vi "Test Overlay Sector.vi"() -> ()   [LabVIEW 2013]
uses:
  Test Sector Cluster.ctl
panel:
  in  "All?":bool
  in  "Sector":u8=3
  out "Image":T1(plugin-control)
  in  "File Path":path
  in  "[Test Sectors]":T2[](array[typedef])=array[43543 elements]
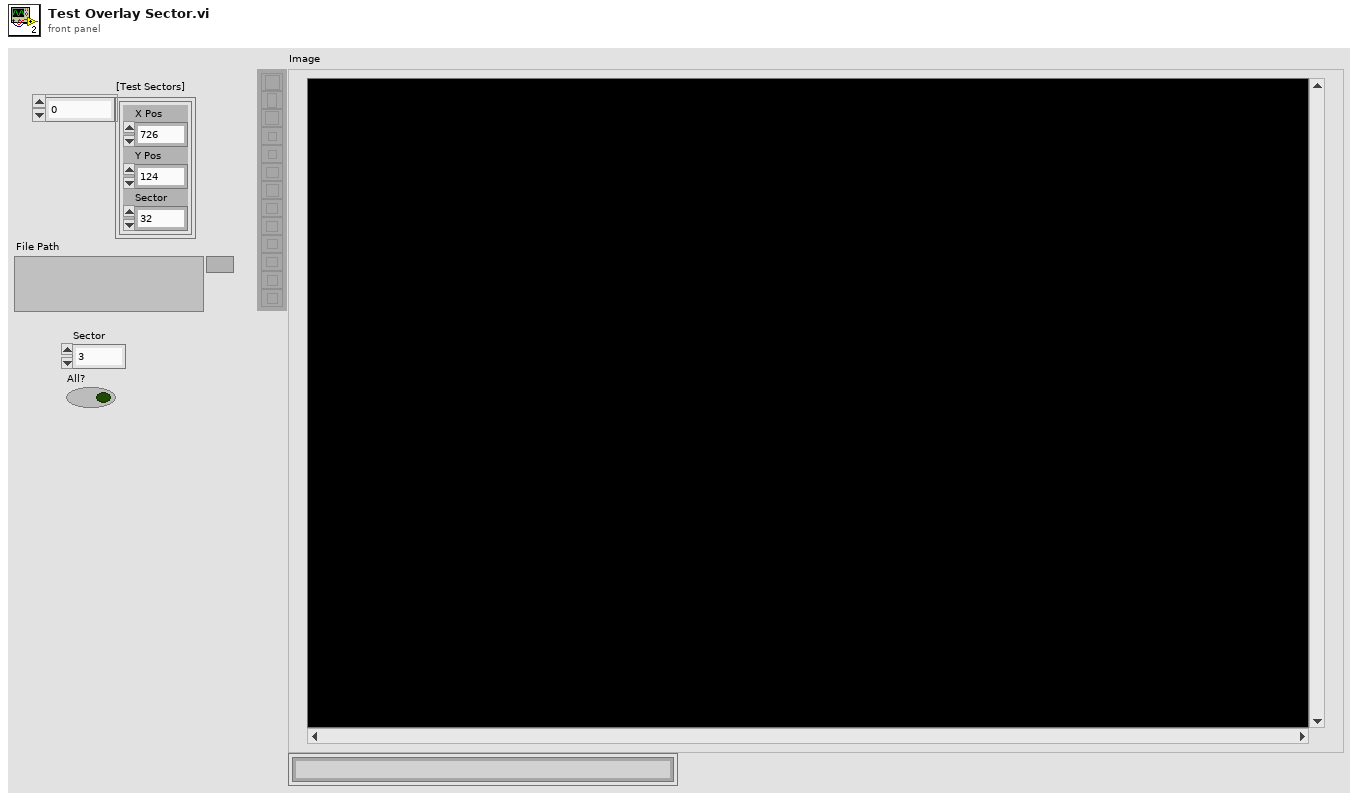
[diagram p1: front panel]
types:
  T1 = typedef "IMAQ Image.ctl" = refnum<image>
  T2 = typedef "Test Sector Cluster.ctl" = cluster{"X Pos":u16, "Y Pos":u16, "Sector":u8}
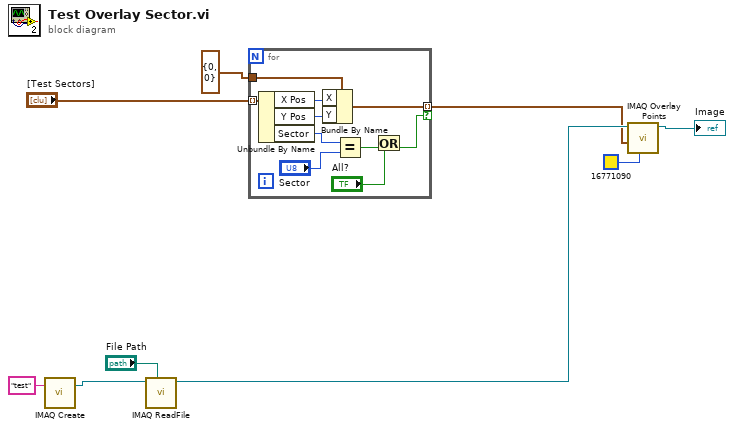
[diagram p0: block diagram]
diagram:
  n1 = call "IMAQ Create"("Image Name"="test") -> ("New Image"=w8:T1)  [unwired: 4 in, 1 out]
  n2 = call "IMAQ ReadFile"("File Path"="File Path", "Image"=w8) -> ("Image Out"=w5:T1)  [unwired: 5 in, 4 out]
  n3 = for {
    tunnel: cluster{"X":i32, "Y":i32} {"X"=0, "Y"=0} ("Point") -> [w19]
    tunnel: "[Test Sectors]" -> [w18] mode=indexing
    tunnel: [w15] -> w3 mode=indexing if=w11
    n4 = Unbundle By Name(w18) -> ("X Pos"=w17:u16, "Y Pos"=w16:u16, "Sector"=w14:u8)
    n5 = Bundle By Name(cluster=w19, "X"=w17, "Y"=w16) -> (w15:cluster{"X":i32, "Y":i32})
    n6 = Equal?(x=w14, y="Sector") -> (x = y?=w12:bool)
    n7 = Or(x="All?", y=w12) -> (x .or. y?=w11:bool)
  }
  n8 = call "IMAQ Overlay Points"("Color"=u32 16771090, "Array of Points"=w3, "Image"=w5) -> ("Image Out"=→"Image":T1)  [unwired: 7 in, 1 out]
